vi "Teleop.vi"(10 "Match Info":T1={"Autonomous Elapsed Seconds"=0.0, "TeleOp Elapsed Seconds"=0.0, "Disabled Elapsed Seconds"=0.0, "Visited Autonomous"=FALSE, "Visited TeleOp"=FALSE, "Visited Disabled"=FALSE, "Autonomous Settings"={"Autonomous Style"=enum."Independent", "VI Refnum"=refnum}}, 11 "Call Context":T2) -> ()   [LabVIEW 2013]
doc: "This VI is called for each TeleOp packet received from the DS where the robot is not disabled. It is often used to read from the joysticks and update I/O or to update setpoints for timed control loops. It should complete and return within 20 milliseconds or it may miss DS packets."
uses:
  <vilib>/Rock Robotics/WPI/DriverStation/WPI_DriverStationDerivedRobotMode.ctl
  <vilib>/Rock Robotics/WPI/DriverStation/WPI_DriverStationMatch Info.ctl
  <vilib>/Rock Robotics/WPI/RobotDrive/WPI_RobotDriveMotorSelectorEnum.ctl
  <vilib>/Rock Robotics/WPI/Relay/WPI_RelayValue.ctl
  Robot Global Data.vi
  <vilib>/Rock Robotics/WPI/Joystick/WPI_JoystickGetSetRefNum.vi
  <vilib>/Rock Robotics/WPI/RobotDrive/WPI_RobotDriveGetSetRefNum.vi
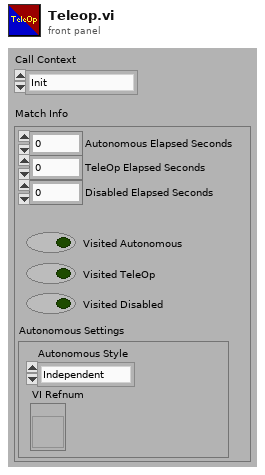
[diagram p1: front panel]
types:
  T1 = typedef "WPI_DriverStationMatch Info.ctl" = cluster{"Autonomous Elapsed Seconds":dbl, "TeleOp Elapsed Seconds":dbl, "Disabled Elapsed Seconds":dbl, "Visited Autonomous":bool, "Visited TeleOp":bool, "Visited Disabled":bool, "Autonomous Settings":cluster{"Autonomous Style":enum16{"Iterative", "Independent"}, "VI Refnum":refnum<vi>}}
  T2 = typedef "WPI_DriverStationDerivedRobotMode.ctl" = enum16{"Init", "Execute", "Stop"}
  T3 = enum16{"Text (00)", "Shoot Status (01)", "Shoot Dist. (02)", "Pressure (03)", "Feed Dist. (04)", "Shutdown (99)"}
  T4 = cluster{"proportional gain (Kc)":dbl, "integral time (Ti, min)":dbl, "derivative time (Td, min)":dbl}
  T5 = typedef "WPI_RobotDriveMotorSelectorEnum.ctl" = enum16{"Rear Left Motor", "Rear Right Motor", "Front Left Motor", "Front Right Motor"}
  T6 = typedef "WPI_RobotDriveDevRef.ctl" = cluster{"DevStatus":errorcluster, "Motors[]":T7[], "Square Inputs":bool, "Max Output":dbl, "Isochronous":bool}
  T7 = typedef "WPI_MotorControlDeviceRef.ctl" = cluster{"DeviceStatus":errorcluster, "Type":enum16{"PWM", "CAN"}, "PWM":cluster{"Digital Module":T8, "PWM Channel":T9, "DeadBand":T10}, "CAN":cluster{"Device Number":u8, "Control Mode":T11, "Semaphore":T12, "Max Vout":dbl}, "Invert":bool, "TransformRef":T13, "InvTransformRef":T13}
  T8 = typedef "FPGA_TypedefDigitalModule.ctl" = enum16{"Digital Module 1", "Digital Module 2"}
  T9 = typedef "FPGA_DIOPWMChannel.ctl" = enum8{"PWM 1", "PWM 2", "PWM 3", "PWM 4", "PWM 5", "PWM 6", "PWM 7", "PWM 8", "PWM 9", "PWM 10", "Invalid"}
  T10 = typedef "WPI_PWMDeadband.ctl" = cluster{"Name":string, "maxPositivePwm":i32, "minPositivePwm":i32, "centerPwm":i32, "maxNegativePwm":i32, "minNegativePwm":i32, "angularRange":u16}
  T11 = typedef "WPI_CANJaguar_ControlMode.ctl" = enum8{"Percent VBus", "Current", "Speed", "Position", "Voltage"}
  T12 = typedef "Semaphore RefNum" = refnum<k1>
  T13 = typedef "WPI_PWMTransform_ConPane.ctl" = refnum<vi>
  T14 = typedef "WPI_JoystickDevRef.ctl" = cluster{"Device":T15}
  T15 = typedef "WPI_JoystickDeviceEnum.ctl" = enum16{"USB 1", "USB 2", "USB 3", "USB 4", "Kinect 1", "Kinect 2"}
  T16 = typedef "WPI_JoystickButtonState.ctl" = cluster{"A":bool, "B":bool, "X":bool, "Y":bool, "L1":bool, "R1":bool, "Select":bool, "Start":bool, "L3":bool, "R3":bool, "Button 11":bool, "Button 12":bool}
  T17 = cluster{"Left Joystick (x)":dbl, "Left Joystick (y)":dbl, "Trigger":dbl, "Right Joystick (x)":dbl, "Right Joystick (y)":dbl, "D-Pad":dbl}
  T18 = typedef "WPI_EncoderDevRef.ctl" = cluster{"DevStatus":errorcluster, "EncoderIndex":T19, "CounterIndex":T20, "DistancePerCount":dbl, "Decoding Type":T21}
  T19 = typedef "FPGA_EncoderIdx.ctl" = enum8{"Enc 0", "Enc 1", "Enc 2", "Enc 3", "Invalid"}
  T20 = typedef "FPGA_CounterCtrSystemIndex.ctl" = enum8{"Ctr 0", "Ctr 1", "Ctr 2", "Ctr 3", "Ctr 4", "Ctr 5", "Ctr 6", "Ctr 7", "Invalid"}
  T21 = typedef "WPI_EncoderType.ctl" = enum16{"1x", "2x", "4x"}
  T22 = cluster{"Motors[]":T18[], "DevStatus":errorcluster, "Max Speed[]":dbl[]}
  T23 = typedef "WPI_GyroDevRef.ctl" = cluster{"DevStatus":errorcluster, "Analog Module":T24, "Analog Channel":T25, "Offset":dbl, "Gain (VoltsPerDegree/Second)":dbl}
  T24 = typedef "FPGA_TypedefAnalogModule.ctl" = enum16{"Analog Module 1", "Analog Module 2"}
  T25 = typedef "FPGA_AIChannel.ctl" = enum8{"AI 1", "AI 2", "AI 3", "AI 4", "AI 5", "AI 6", "AI 7", "AI 8", "Invalid"}
  T26 = typedef "WPI_RelayValue.ctl" = enum16{"Off", "On", "Forward", "Reverse"}
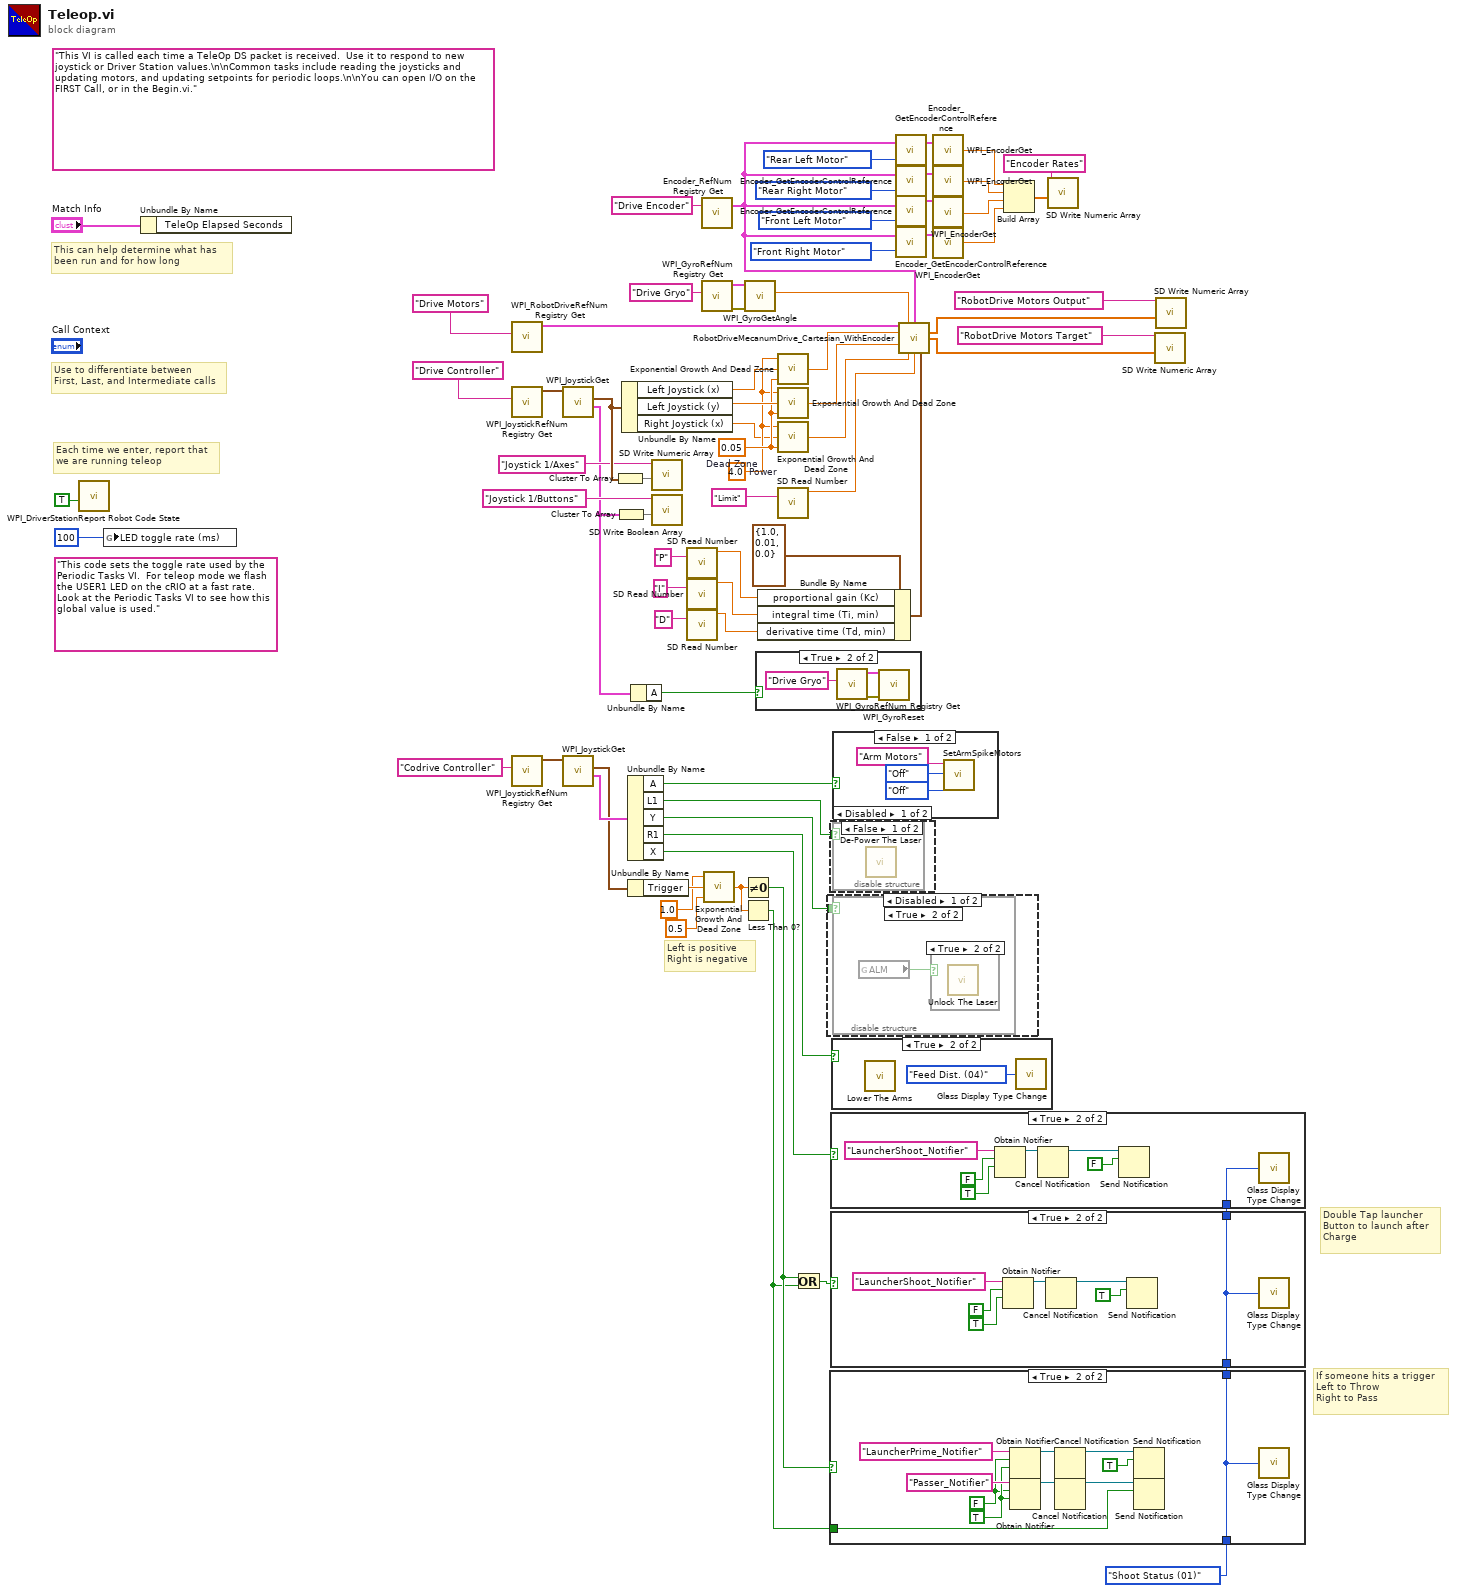
[diagram p0: block diagram]
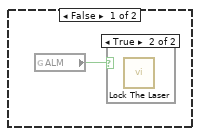
[diagram p2: hidden frame]
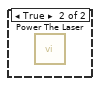
[diagram p9: hidden frame]
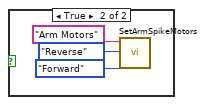
[diagram p11: hidden frame]
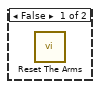
[diagram p12: hidden frame]
diagram:
  w58 = 4.0  # Power
  w59 = 0.05  # Dead Zone
  (unwired) "This code sets the toggle rate used by the Periodic Tasks VI.  For teleop mode we flash the USER1 LED on the cRIO at a fast rate.  Look at the Periodic Tasks VI to see how this global value is used."
  (unwired) "This VI is called each time a TeleOp DS packet is received.  Use it to respond to new joystick or Driver Station values.\n\nCommon tasks include reading the joysticks and updating motors, and updating setpoints for periodic loops.\n\nYou can open I/O on the FIRST Call, or in the Begin.vi."
  # "Double Tap launcher\nButton to launch after\nCharge"
  # "If someone hits a trigger \nLeft to Throw\nRight to Pass"
  # "Left is positive\nRight is negative"
  # "Each time we enter, report that\nwe are running teleop"
  # "Use to differentiate between\nFirst, Last, and Intermediate calls"
  # "This can help determine what has\nbeen run and for how long"
  n1 = call <vilib>:"WPI_DriverStationReport Robot Code State.vi"("TeleOp"=TRUE ("Autonomous")) -> ()  [unwired: 10 in, 1 out]
  n2 = global write "Robot Global Data.vi" "LED toggle rate (ms)"(u32 100 ("LED ms toggle rate")) -> ()
  n3 = Unbundle By Name("Match Info") -> ()  [unwired: 1 out]
  n4 = call <vilib>:"WPI_RobotDriveRefNum Registry Get.vi"("refnum name"="Drive Motors") -> ("RobotDriveDevRef"=w73:T6)  [unwired: 1 in, 9 out]
  n5 = call <vilib>:"WPI_JoystickRefNum Registry Get.vi"("refnum name"="Drive Controller") -> ("JoystickDevRef"=w71:T14)  [unwired: 1 in, 9 out]
  n6 = call <vilib>:"WPI_JoystickRefNum Registry Get.vi"("refnum name"="Codrive Controller") -> ("JoystickDevRef"=w20:T14)  [unwired: 9 in, 1 out]
  n7 = call <vilib>:"WPI_JoystickGet.vi"("JoystickDevRef"=w71) -> ("Buttons"=w18:T16, "Axes"=w66:T17)  [unwired: 1 in, 4 out]
  n8 = call <vilib>:"WPI_JoystickGet.vi"("JoystickDevRef"=w20) -> ("Buttons"=w15:T16, "Axes"=w12:T17)  [unwired: 4 in, 1 out]
  n9 = Cluster To Array(cluster=w66) -> (array=w65:dbl[])
  n10 = Cluster To Array(cluster=w18) -> (array=w68:bool[])
  n11 = Unbundle By Name(w66) -> ("Left Joystick (x)"=w60:dbl, "Left Joystick (y)"=w61:dbl, "Right Joystick (x)"=w16:dbl)
  n12 = Unbundle By Name(w15) -> ("A"=w19:bool, "L1"=w17:bool, "Y"=w13:bool, "R1"=w14:bool, "X"=w5:bool)
  n13 = Unbundle By Name(w12) -> ("Trigger"=w11:dbl)
  n14 = Unbundle By Name(w18) -> ("A"=w53:bool)
  n15 = call <vilib>:"SD Write Numeric Array.vi"("Numeric Array"=w65, "Name"="Joystick 1/Axes") -> ()  [unwired: 8 in, 2 out]
  n16 = call <vilib>:"SD Write Boolean Array.vi"("Boolean Array"=w68, "Name"="Joystick 1/Buttons") -> ()  [unwired: 8 in, 2 out]
  n17 = call <vilib>:"SD Read Number.vi"("Name"="P") -> ("Numeric"=w30:dbl)  [unwired: 8 in, 2 out]
  n18 = call <vilib>:"SD Read Number.vi"("Name"="I") -> ("Numeric"=w29:dbl)  [unwired: 8 in, 2 out]
  n19 = call <vilib>:"SD Read Number.vi"("Name"="D") -> ("Numeric"=w22:dbl)  [unwired: 8 in, 2 out]
  n20 = call "Encoder_RefNum Registry Get.vi"("refnum name"="Drive Encoder") -> ("RobotEncoderRef Out"=w36:T22)  [unwired: 1 in, 1 out]
  n21 = call <vilib>:"WPI_GyroRefNum Registry Get.vi"("refnum name"="Drive Gryo") -> ("error out"=w57:errorcluster, "GyroDevRef"=w56:T23)  [unwired: 9 in]
  n22 = call "Exponential Growth And Dead Zone.vi"("Dead Zone"=0.5, "Joy Stick Input"=w11, "Power"=1.0) -> ("Fixed Output"=w8:dbl)
  n23 = Not Equal To 0?(x=w8) -> (x != 0?=w7:bool)
  n24 = Less Than 0?(x=w8) -> (x < 0?=w6:bool)
  n25 = call <vilib>:"WPI_GyroGetAngle.vi"("error in (no error)"=w57, "GyroDevRef"=w56) -> ("Angle"=w55:dbl)  [unwired: 6 in, 3 out]
  n26 = case shown="True" w53 {
    frame False {
    }
    frame True {
      n27 = call <vilib>:"WPI_GyroRefNum Registry Get.vi"("refnum name"="Drive Gryo") -> ("error out"=w78:errorcluster, "GyroDevRef"=w77:T23)  [unwired: 9 in]
      n28 = call <vilib>:"WPI_GyroReset.vi"("error in (no error)"=w78, "GyroDevRef"=w77) -> ()  [unwired: 8 in, 2 out]
    }
  }
  n29 = Bundle By Name(cluster=T4 {"proportional gain (Kc)"=1.0, "integral time (Ti, min)"=0.01, "derivative time (Td, min)"=0.0} ("PID gains"), "proportional gain (Kc)"=w30, "integral time (Ti, min)"=w29, "derivative time (Td, min)"=w22) -> (w28:T4)
  n30 = call "Exponential Growth And Dead Zone.vi"("Dead Zone"=w59, "Joy Stick Input"=w60, "Power"=w58) -> ("Fixed Output"=w24:dbl)
  n31 = call "Exponential Growth And Dead Zone.vi"("Dead Zone"=w59, "Joy Stick Input"=w61, "Power"=w58) -> ("Fixed Output"=w23:dbl)
  n32 = call "Exponential Growth And Dead Zone.vi"("Dead Zone"=w59, "Joy Stick Input"=w16, "Power"=w58) -> ("Fixed Output"=w25:dbl)
  n33 = call <vilib>:"SD Read Number.vi"("Name"="Limit") -> ("Numeric"=w35:dbl)  [unwired: 8 in, 2 out]
  n34 = Or(x=w7, y=w6) -> (x .or. y?=w4:bool)
  n35 = disable-structure shown="Disabled" {
    disable-tunnel: w13 -> [w79 _]
    frame Disabled {
      n36 = case shown="True" w79 {
        frame False {
          n37 = global read "Robot Global Data.vi" "ALM"() -> (w80:bool)
          n38 = case shown="True" w80 {
            frame False {
            }
            frame True {
              n39 = call "Lock The Laser.vi"() -> ()  [unwired: 12 in]
            }
          }
        }
        frame True {
          n40 = global read "Robot Global Data.vi" "ALM"() -> (w81:bool)
          n41 = case shown="True" w81 {
            frame False {
            }
            frame True {
              n42 = call "Unlock The Laser.vi"() -> ()  [unwired: 12 in]
            }
          }
        }
      }
    }
    frame Enabled {
    }
  }
  n43 = case shown="True" w7 {
    tunnel: w6 -> [_ w89]
    tunnel: [_ w82] -> w2
    tunnel: T3."Shoot Status (01)" ("Data To Glass Type") -> [_ w82]
    frame False {
    }
    frame True {
      w88 = TRUE
      w87 = FALSE
      n44 = Obtain Notifier(name (unnamed)="LauncherPrime_Notifier", notification data type=w87, create if not found? (T)=w88) -> (notifier out=w86:refnum<notifier>)  [unwired: 1 in, 2 out]
      n45 = Obtain Notifier(name (unnamed)="Passer_Notifier", notification data type=w87, create if not found? (T)=w88) -> (notifier out=w84:refnum<notifier>)  [unwired: 1 in, 2 out]
      n46 = Cancel Notification(0:w86) -> (8:w85:refnum<notifier>)  [unwired: 1 in, 2 out]
      n47 = Cancel Notification(0:w84) -> (8:w83:refnum<notifier>)  [unwired: 1 in, 2 out]
      n48 = Send Notification(notification=TRUE, notifier=w85) -> ()  [unwired: 1 in, 2 out]
      n49 = Send Notification(notification=w89, notifier=w83) -> ()  [unwired: 1 in, 2 out]
      n50 = call "Glass Display Type Change.vi"("Data To Glass Type"=w82) -> ()
    }
  }
  n51 = disable-structure shown="Disabled" {
    disable-tunnel: w17 -> [w93 _]
    frame Disabled {
      n52 = case shown="False" w93 {
        frame False {
          n53 = call "De-Power The Laser.vi"() -> ()  [unwired: 12 in]
        }
        frame True {
          n54 = call "Power The Laser.vi"() -> ()  [unwired: 12 in]
        }
      }
    }
    frame Enabled {
    }
  }
  n55 = case shown="True" w4 {
    tunnel: [_ w94] -> w3
    tunnel: w2 -> [_ w94]
    frame False {
    }
    frame True {
      n56 = Obtain Notifier(name (unnamed)="LauncherShoot_Notifier", notification data type=FALSE, create if not found? (T)=TRUE) -> (notifier out=w96:refnum<notifier>)  [unwired: 1 in, 2 out]
      n57 = Cancel Notification(0:w96) -> (8:w95:refnum<notifier>)  [unwired: 1 in, 2 out]
      n58 = Send Notification(notification=TRUE, notifier=w95) -> ()  [unwired: 1 in, 2 out]
      n59 = call "Glass Display Type Change.vi"("Data To Glass Type"=w94) -> ()
    }
  }
  n60 = case shown="True" w5 {
    tunnel: w3 -> [_ w101]
    frame False {
    }
    frame True {
      n61 = Obtain Notifier(name (unnamed)="LauncherShoot_Notifier", notification data type=FALSE, create if not found? (T)=TRUE) -> (notifier out=w103:refnum<notifier>)  [unwired: 1 in, 2 out]
      n62 = Cancel Notification(0:w103) -> (8:w102:refnum<notifier>)  [unwired: 1 in, 2 out]
      n63 = Send Notification(notification=FALSE, notifier=w102) -> ()  [unwired: 1 in, 2 out]
      n64 = call "Glass Display Type Change.vi"("Data To Glass Type"=w101) -> ()
    }
  }
  n65 = case shown="True" w14 {
    frame False {
      n66 = call "Reset The Arms.vi"() -> ()  [unwired: 12 in]
    }
    frame True {
      n67 = call "Lower The Arms.vi"() -> ()  [unwired: 12 in]
      n68 = call "Glass Display Type Change.vi"("Data To Glass Type"=T3."Feed Dist. (04)") -> ()
    }
  }
  n69 = case shown="False" w19 {
    frame False {
      n70 = call "SetArmSpikeMotors.vi"("Direction For Right"=WPI_RelayValue."Off", "Direction For Left"=WPI_RelayValue."Off", "Name"="Arm Motors") -> ()  [unwired: 8 in, 1 out]
    }
    frame True {
      n71 = call "SetArmSpikeMotors.vi"("Direction For Right"=WPI_RelayValue."Forward", "Direction For Left"=WPI_RelayValue."Reverse", "Name"="Arm Motors") -> ()  [unwired: 8 in, 1 out]
    }
  }
  n72 = call "Encoder_GetEncoderControlReference.vi"("MotorIndex"=WPI_RobotDriveMotorSelectorEnum."Rear Left Motor", "RobotEncoderRef"=w36) -> ("EncoderDevRef"=w41:T18)  [unwired: 1 out]
  n73 = call "Encoder_GetEncoderControlReference.vi"("MotorIndex"=WPI_RobotDriveMotorSelectorEnum."Rear Right Motor", "RobotEncoderRef"=w36) -> ("EncoderDevRef"=w42:T18)  [unwired: 1 out]
  n74 = call "Encoder_GetEncoderControlReference.vi"("MotorIndex"=WPI_RobotDriveMotorSelectorEnum."Front Left Motor", "RobotEncoderRef"=w36) -> ("EncoderDevRef"=w43:T18)  [unwired: 1 out]
  n75 = call "Encoder_GetEncoderControlReference.vi"("MotorIndex"=WPI_RobotDriveMotorSelectorEnum."Front Right Motor", "RobotEncoderRef"=w36) -> ("EncoderDevRef"=w44:T18)  [unwired: 1 out]
  n76 = call "RobotDriveMecanumDrive_Cartesian_WithEncoder.vi"("RobotDriveDevRef"=w73, "Gyro Angle"=w55, "RobotEncoderRef"=w36, "X"=w24, "Y"=w23, "Rotation"=w25, "Limit"=w35, "PID gains"=w28) -> ("Motor Values"=w62:dbl[], "Target Values"=w26:dbl[])  [unwired: 4 in, 2 out]
  n77 = call <vilib>:"WPI_EncoderGet.vi"("EncoderDevRef"=w41) -> ("Rate"=w50:dbl)  [unwired: 5 in, 5 out]
  n78 = call <vilib>:"WPI_EncoderGet.vi"("EncoderDevRef"=w42) -> ("Rate"=w47:dbl)  [unwired: 5 in, 5 out]
  n79 = call <vilib>:"WPI_EncoderGet.vi"("EncoderDevRef"=w43) -> ("Rate"=w49:dbl)  [unwired: 5 in, 5 out]
  n80 = call <vilib>:"WPI_EncoderGet.vi"("EncoderDevRef"=w44) -> ("Rate"=w48:dbl)  [unwired: 5 in, 5 out]
  n81 = Build Array(w50, w47, w49, w48) -> (w46:dbl[])
  n82 = call <vilib>:"SD Write Numeric Array.vi"("Numeric Array"=w46, "Name"="Encoder Rates") -> ()  [unwired: 8 in, 2 out]
  n83 = call <vilib>:"SD Write Numeric Array.vi"("Numeric Array"=w26, "Name"="RobotDrive Motors Target") -> ()  [unwired: 8 in, 2 out]
  n84 = call <vilib>:"SD Write Numeric Array.vi"("Numeric Array"=w62, "Name"="RobotDrive Motors Output") -> ()  [unwired: 8 in, 2 out]
